vi "Open PDF File LV2016.vi"(7 "error in (no error)":errorcluster, 8 "Pdf file path":path) -> (1 "error out":errorcluster)   [LabVIEW 2016]
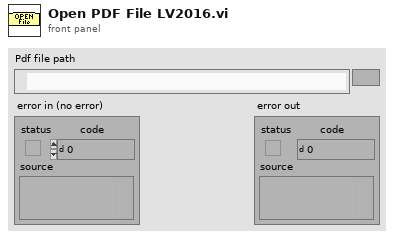
[diagram p1: front panel]
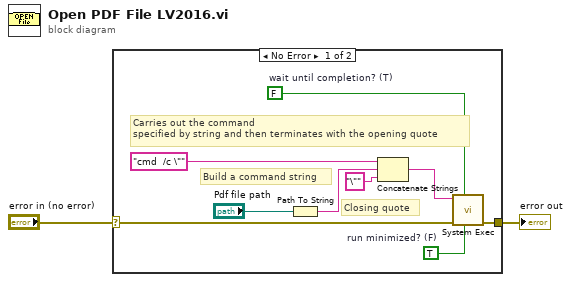
[diagram p0: block diagram]
diagram:
  n1 = case shown="No Error" "error in (no error)" {
    selector: "error in (no error)" -> [w4 w12]
    tunnel: [w3 w12] -> w1
    frame No Error {
      w6 = TRUE  # run minimized? (F)
      w5 = FALSE  # wait until completion? (T)
      # "Build a command string"
      # "Closing quote"
      # "Carries out the command \nspecified by string and then terminates with the opening quote"
      n2 = Path To String(path="Pdf file path") -> (string=w10:string)
      n3 = Concatenate Strings("cmd  /c \"", w10, "\"") -> (w8:string)
      n4 = call <vilib>:"System Exec.vi"("run minimized? (F)"=w6, "wait until completion? (T)"=w5, "error in (no error)"=w4, "command line"=w8) -> ("error out"=w3:errorcluster)  [unwired: 2 in, 5 out]
    }
    frame Error {
    }
  }
  "error out" <- w1
